vi "Get Area Temperature.vi"(8 "error in (no error)":errorcluster, 10 "Area":T1, 11 "Optris PI in":refnum<class "Optris PI.lvclass">) -> (0 "error out":errorcluster, 1 "Avg Temp":dbl, 2 "Area Temps":dbl[][](array[numeric]), 3 "Optris PI out":refnum<class "Optris PI.lvclass">)   [LabVIEW 2018, in "Optris PI.lvlib" / "Optris PI.lvclass"]
uses:
  Optris PI.lvclass
  PPLs/Thermal Camera/Parent/Thermal Camera.lvlibp/Accessors/Area Coordinates.ctl
  Optris PI.lvclass/Optris PI.ctl
  <instrlib>/Optris PI/libirimager_direct_binding.lvlib
  PPLs/Thermal Camera/Parent/Thermal Camera.lvlibp/Thermal Camera.lvclass
  C:/AME Test Engineering/LabVIEW/PPLs/Thermal Camera/Parent/Thermal Camera.lvlibp/Thermal Camera.lvclass
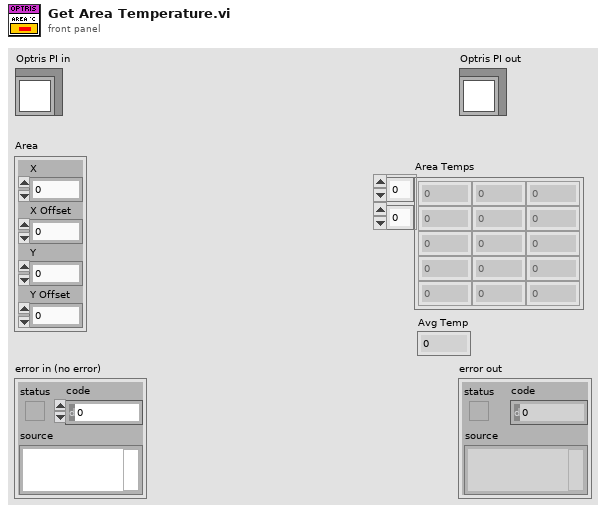
[diagram p1: front panel]
types:
  T1 = typedef "Thermal Camera.lvlibp/Thermal Camera.lvclass/Area Coordinates.ctl" = cluster{"X":i32, "X Offset":i32, "Y":i32, "Y Offset":i32}
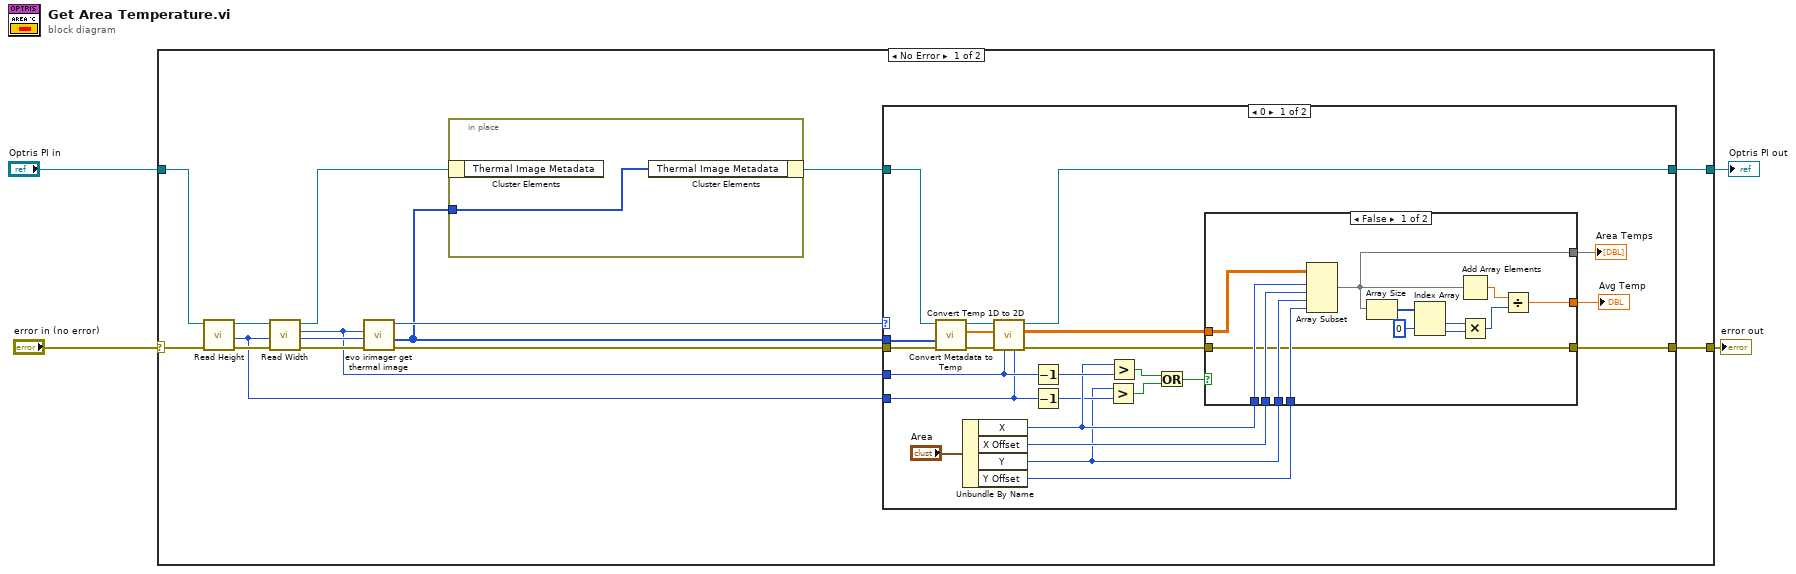
[diagram p0: block diagram]
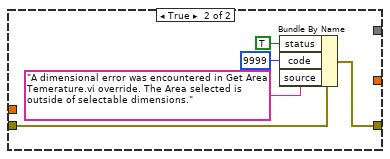
[diagram p2: hidden frame]
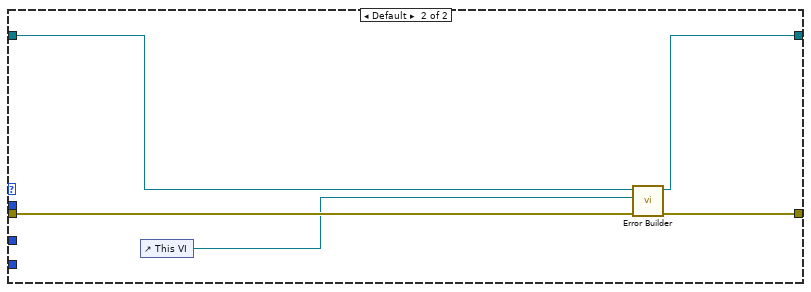
[diagram p3: hidden frame]
diagram:
  n1 = case shown="No Error" "error in (no error)" {
    selector: "error in (no error)" -> [w17 w68]
    tunnel: [w11 w69] -> w3
    tunnel: "Optris PI in" -> [w18 w69]
    tunnel: [w10 w68] -> w1
    frame No Error {
      n2 = call "Read Height.vi"("error in (no error)"=w17, "Thermal Camera in"=w18) -> ("error out"=w15:errorcluster, "Height"=w9:u32, "Thermal Camera out"=w16:refnum<class "Optris PI.lvclass">)  [unwired: 7 in]
      n3 = call "Read Width.vi"("error in (no error)"=w15, "Thermal Camera in"=w16) -> ("error out"=w14:errorcluster, "Width"=w8:u32, "Thermal Camera out"=w7:refnum<class "Optris PI.lvclass">)  [unwired: 7 in]
      n4 = call <instrlib>:"evo irimager get thermal image.vi"("error in (no error)"=w14, "h"=w9, "w"=w8) -> ("error out"=w12:errorcluster, "data out"=w5:u16[], "function return"=w13:i32)  [unwired: 4 in, 2 out]
      n5 = in-place {
        in-place-border: w5 -> [w19]
        n6 = in-place-cluster #1(w7) -> ()  [unwired: 1 out]
        n7 = in-place-cluster #1("Thermal Image Metadata"=w19) -> (w6:refnum<class "Optris PI.lvclass">)
      }
      n8 = case shown="0" w13 {
        tunnel: w12 -> [w42 w67]
        tunnel: w6 -> [w43 w65]
        tunnel: [w37 w64] -> w11
        tunnel: [w21 w63] -> w10
        tunnel: w5 -> [w41 _]
        tunnel: w9 -> [w30 _]
        tunnel: w8 -> [w31 _]
        frame 0 {
          n9 = call "Convert Metadata to Temp.vi"("error in (no error)"=w42, "Temp Metadata"=w41, "Optris PI in"=w43) -> ("error out"=w38:errorcluster, "Temperatures (Def. C)"=w40:dbl[], "Optris PI out"=w39:refnum<class "Optris PI.lvclass">)  [unwired: 6 in]
          n10 = Unbundle By Name("Area") -> ("X"=w28:i32, "X Offset"=w34:i32, "Y"=w26:i32, "Y Offset"=w33:i32)
          n11 = call "Convert Temp 1D to 2D.vi"("Width"=w31, "Height"=w30, "error in (no error)"=w38, "Temperatures (C)"=w40, "Optris PI in"=w39) -> ("error out"=w22:errorcluster, "Area Temps"=w36:dbl[][], "Optris PI out"=w37:refnum<class "Optris PI.lvclass">)  [unwired: 4 in]
          n12 = Decrement(x=w31) -> (x-1=w29:u32)
          n13 = Decrement(x=w30) -> (x-1=w27:u32)
          n14 = Greater?(x=w26, y=w27) -> (0:w24:bool)
          n15 = Greater?(x=w28, y=w29) -> (0:w25:bool)
          n16 = Or(x=w25, y=w24) -> (x .or. y?=w23:bool)
          n17 = case shown="False" w23 {
            tunnel: w36 -> [w57 _]
            tunnel: w34 -> [w56 _]
            tunnel: w33 -> [w55 _]
            tunnel: [w51 _] -> w32
            tunnel: w28 -> [w54 _]
            tunnel: w26 -> [w53 _]
            tunnel: w22 -> [w52 w62]
            tunnel: [w52 w58] -> w21
            tunnel: [w44 _] -> w20
            frame False {
              n18 = Array Subset(array=w57, index (row)=w54, length (row)=w56, index (col)=w53, length (col)=w55) -> (w51:dbl[][])
              n19 = Array Size(array=w51) -> (size(s)=w50:i32[])
              n20 = Index Array(array=w50, index #1=0 ("index")) -> (element #1=w47:i32, element #2=w48:i32)  [unwired: 1 in]
              n21 = Add Array Elements(numeric array=w51) -> (sum=w46:dbl)
              n22 = Multiply(x=w47, y=w48) -> (x*y=w45:i32)
              n23 = Divide(x=w46, y=w45) -> (x/y=w44:dbl)
            }
            frame True {
              n24 = Bundle By Name(cluster=w62, "status"=TRUE, "code"=9999, "source"="A dimensional error was encountered in Get Area Temerature.vi override. The Area selected is outside of selectable dimensions.") -> (w58:errorcluster)
            }
          }
          "Area Temps" <- w32
          "Avg Temp" <- w20
        }
        frame Default {
          n25 = control-ref of="This VI"() -> (w66:refnum<vi>)
          n26 = call "Error Builder.vi"("error in (no error)"=w67, "This VI"=w66, "Optris PI in"=w65) -> ("Error out"=w63:errorcluster, "Optris PI out"=w64:refnum<class "Optris PI.lvclass">)  [unwired: 7 in]
        }
      }
    }
    frame Error {
    }
  }
  "error out" <- w1
  "Optris PI out" <- w3
